vi "SubVI_MODCA.vi"(11 "Points":i32=10) -> (3 "Disorder Pattern":dbl[](graph))   [LabVIEW 2019]
panel:
  in  "Set":bool
  in  "Generate":bool
  in  "App":dbl=0.1
  in  "Step width":dbl=0.2
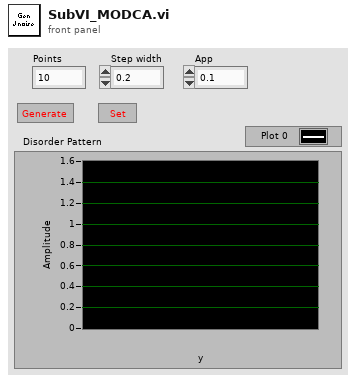
[diagram p1: front panel]
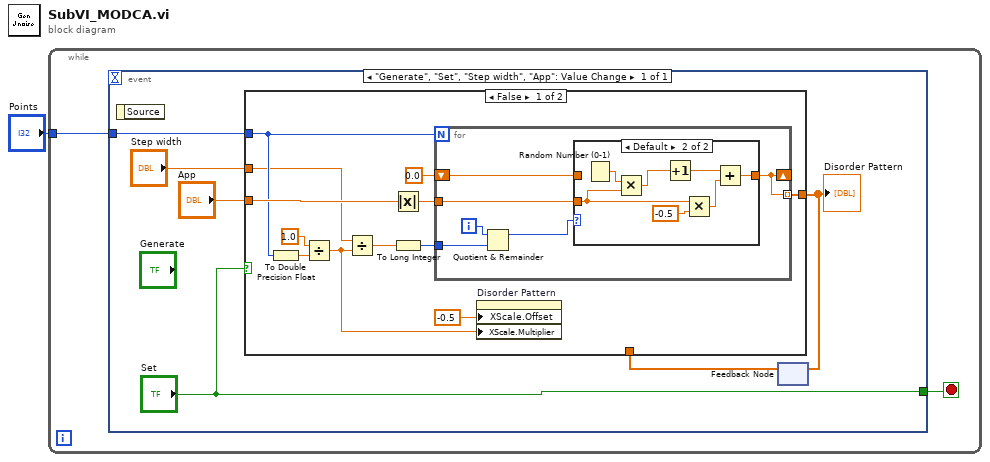
[diagram p0: block diagram]
diagram:
  n1 = while {
    tunnel: "Points" -> [w2]
    stop <- w3 stop-if-true
    n2 = event shown="[0] \"Generate\", \"Set\", \"Step width\", \"App\": Value Change" {
      selector: _ -> [_]
      dyn-events: _ -> [_]
      timeout: _ -> [_]
      tunnel: ["Set"] -> w3
      tunnel: w2 -> [w5]
      event "Generate", "Set", "Step width", "App": Value Change {
        n3 = event-data() -> ()  [unwired: 1 in, 1 out]
        n4 = feedback #1() -> (w6:dbl[])  [unwired: 1 in]
        n5 = case shown="False" "Set" {
          tunnel: "App" -> [w20 _]
          tunnel: w5 -> [w18 _]
          tunnel: "Step width" -> [w16 _]
          tunnel: [w12 w36] -> w7
          tunnel: w6 -> [_ w36]
          frame False {
            n6 = To Double Precision Float(number=w18) -> (double precision float=w15:dbl)
            n7 = Divide(x=1.0, y=w15) -> (x/y=w10:dbl)
            n8 = Divide(x=w16, y=w10) -> (x/y=w17:dbl)
            n9 = Absolute Value(x=w20) -> (abs(x)=w21:dbl)
            n10 = To Long Integer(number=w17) -> (32bit integer=w19:i32)
            n11 = for {
              N: w18 -> [_]
              tunnel: w19 -> [w26]
              tunnel: w21 -> [w25]
              shift-right: [w23] -> _
              shift-left: 0.0 -> [w24]
              tunnel: [w23] -> w12 mode=indexing
              i -> [w27]
              n12 = Quotient & Remainder(x=w27, y=w26) -> (x-y*floor(x/y)=w22:i32)  [unwired: 1 out]
              n13 = case shown="Default" w22 {
                tunnel: w25 -> [_ w33]
                tunnel: [w28 w29] -> w23
                tunnel: w24 -> [w28 _]
                frame 0 {
                }
                frame Default {
                  n14 = Random Number (0-1)() -> (number: 0 to 1=w35:dbl)
                  n15 = Multiply(x=w35, y=w33) -> (x*y=w34:dbl)
                  n16 = Increment(x=w34) -> (x+1=w31:dbl)
                  n17 = Multiply(x=w33, y=-0.5) -> (x*y=w30:dbl)
                  n18 = Add(x=w31, y=w30) -> (x+y=w29:dbl)
                }
              }
            }
            n19 = property on="Disorder Pattern" class="WFGraph (strict)"("XScale.Offset"=-0.5, "XScale.Multiplier"=w10) -> ()  [unwired: 2 in, 2 out]
          }
          frame True {
          }
        }
        "Disorder Pattern" <- w7
        n20 = feedback-in #1(w7) -> ()
      }
    }
  }
